vi "filter_x.vi"(9 "y":dbl[](array[numeric]), 10 "x":dbl[](array[numeric]), 11 "exclude_where_x":dbl) -> (1 "filtered_y":dbl[](array[numeric]), 2 "filtered_x":dbl[](array[numeric]))   [LabVIEW 2017, in "tools.lvlib"]
uses:
  tools.lvlib
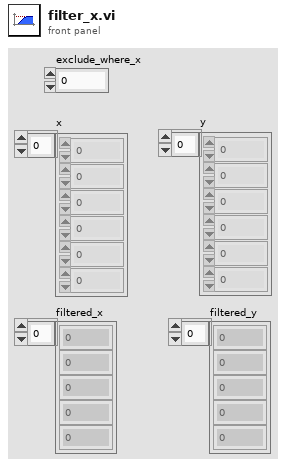
[diagram p1: front panel]
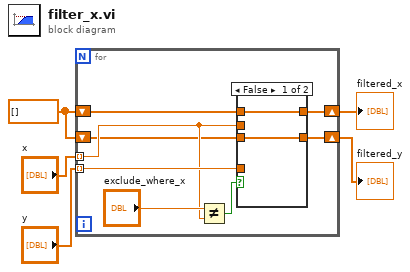
[diagram p0: block diagram]
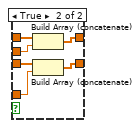
[diagram p2: hidden frame]
diagram:
  w3 = dbl[] [] ("x")
  n1 = for {
    tunnel: "x" -> [w11] mode=indexing
    tunnel: "y" -> [w12] mode=indexing
    shift-right: [w9] -> w2
    shift-left: w3 -> [w10]
    shift-right: [w7] -> w1
    shift-left: w3 -> [w8]
    n2 = Not Equal?(x="exclude_where_x", y=w11) -> (x != y?=w6:bool)
    n3 = case shown="False" w6 {
      tunnel: w12 -> [_ w18]
      tunnel: w11 -> [_ w19]
      tunnel: w10 -> [w15 w21]
      tunnel: [w15 w20] -> w9
      tunnel: w8 -> [w14 w17]
      tunnel: [w14 w16] -> w7
      frame False {
      }
      frame True {
        n4 = Build Array (concatenate)(w21, w19) -> (w20:dbl[])
        n5 = Build Array (concatenate)(w17, w18) -> (w16:dbl[])
      }
    }
  }
  "filtered_x" <- w2
  "filtered_y" <- w1
